vi "Unknown.vi"   [LabVIEW 2018]
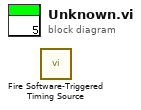
[diagram p0: block diagram]
diagram:
  n1 = call <vilib>:"Fire Software-Triggered Timing Source.vi"() -> ()  [unwired: 10 in, 2 out]
